vi "REST API Example - 1.vi"() -> ()   [LabVIEW 2023, in "LabVIEW LLM.lvlib"]
uses:
  LabVIEW LLM.lvlib
  <vilib>/httpClient/POSTBuffer.vi
  <vilib>/httpClient/LabVIEWHTTPClient.lvlib
panel:
  out "error out":errorcluster
  out "JSON应答":string
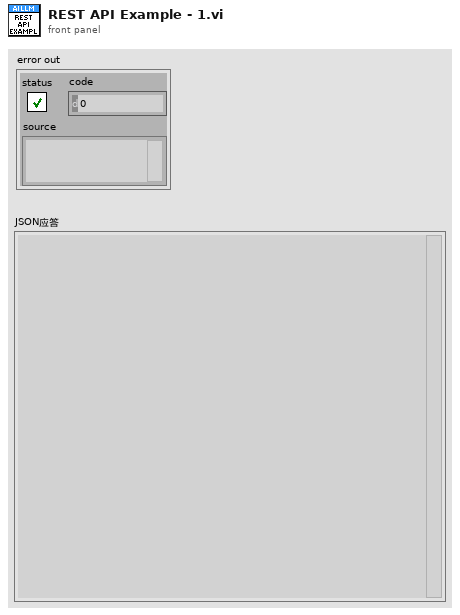
[diagram p1: front panel]
types:
  T1 = typedef "LabVIEWHTTPClient.lvlib/ClientHandle.ctl" = refnum<k1>
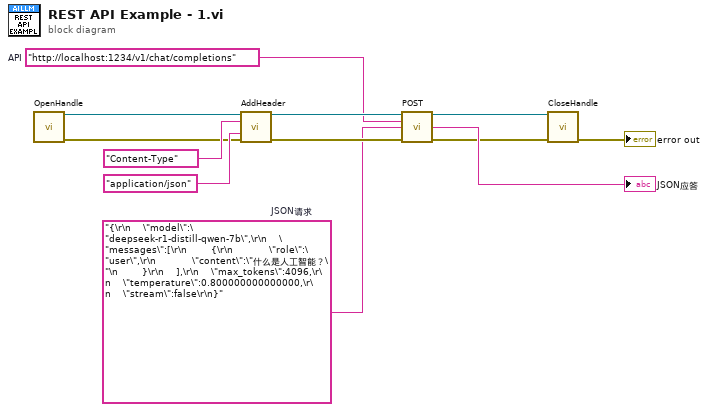
[diagram p0: block diagram]
diagram:
  w1 = "{\r\n    \"model\":\"deepseek-r1-distill-qwen-7b\",\r\n    \"messages\":[\r\n        {\r\n            \"role\":\"user\",\r\n            \"content\":\"什么是人工智能？\"\n        }\r\n    ],\r\n    \"max_tokens\":4096,\r\n    \"temperature\":0.800000000000000,\r\n    \"stream\":false\r\n}"  # JSON请求
  w8 = "http://localhost:1234/v1/chat/completions"  # API
  n1 = call <vilib>:"OpenHandle.vi"() -> ("client handle out"=w7:T1, "error out"=w6:errorcluster)  [unwired: 14 in]
  n2 = call <vilib>:"AddHeader.vi"("client handle"=w7, "header"="Content-Type", "value"="application/json", "error in (no error)"=w6) -> ("client handle out"=w10:T1, "error out"=w9:errorcluster)  [unwired: 10 in]
  n3 = call-poly <vilib>:"POST.vi"("client handle"=w10, "url"=w8, "buffer"=w1, "error in (no error)"=w9) -> ("client handle out"=w4:T1, "body"=→"JSON应答":string, "error out"=w3:errorcluster)  [unwired: 8 in, 1 out]
  n4 = call <vilib>:"CloseHandle.vi"("client handle"=w4, "error in (no error)"=w3) -> ("error out"=→"error out":errorcluster)  [unwired: 13 in]
